vi "Scale 2-Exp Parameter Constraints.vi"(9 "Normalization Factor":dbl, 11 "parameter bounds in":T1) -> (3 "parameter bounds out":T1)   [LabVIEW 2021, in "Fits.lvlib"]
uses:
  Fits.lvlib
  IRF(X)PSED/Decay Fit Parameters In List.ctl
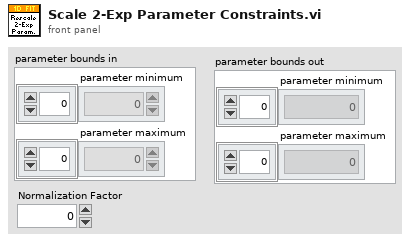
[diagram p1: front panel]
types:
  T1 = cluster{"parameter minimum":dbl[], "parameter maximum":dbl[]}
  T2 = typedef "Fits.lvlib/Decay Fit Parameters In List.ctl" = enum16{"Offset", "Baseline", "A_1", "tau_1", "A_2", "tau_2"}
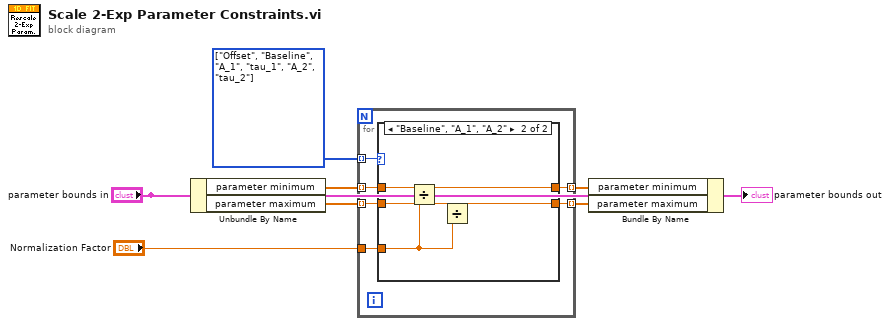
[diagram p0: block diagram]
diagram:
  w7 = T2[] [enum."Offset", enum."Baseline", enum."A_1", enum."tau_1", enum."A_2", enum."tau_2"] items=["Offset", "Baseline", "A_1", "tau_1", "A_2", "tau_2"] ("data")
  n1 = Unbundle By Name("parameter bounds in") -> ("parameter minimum"=w8:dbl[], "parameter maximum"=w5:dbl[])
  n2 = for {
    tunnel: w8 -> [w12] mode=indexing
    tunnel: w7 -> [w14] mode=indexing
    tunnel: "Normalization Factor" -> [w13]
    tunnel: w5 -> [w11] mode=indexing
    tunnel: [w10] -> w3 mode=indexing
    tunnel: [w9] -> w2 mode=indexing
    n3 = case shown="\"Baseline\", \"A_1\", \"A_2\"" w14 {
      tunnel: w13 -> [_ w19]
      tunnel: w12 -> [w16 w21]
      tunnel: w11 -> [w15 w20]
      tunnel: [w16 w17] -> w10
      tunnel: [w15 w18] -> w9
      frame "Offset", Default {
      }
      frame "Baseline", "A_1", "A_2" {
        n4 = Divide(x=w21, y=w19) -> (x/y=w17:dbl)
        n5 = Divide(x=w20, y=w19) -> (x/y=w18:dbl)
      }
    }
  }
  n6 = Bundle By Name(cluster="parameter bounds in", "parameter minimum"=w3, "parameter maximum"=w2) -> (→"parameter bounds out":T1)
